vi "读取配置信息 (子VI).vi"(8 "error in (no error)":errorcluster caption="错误输入（无错误）") -> (0 "错误输出":errorcluster)   [LabVIEW 2022 SP3, in "流量计集成.lvlib"]
uses:
  <vilib>/Utility/config.llb/NI_LVConfig.lvlib
  <userlib>/_OpenG.lib/variantconfig/variantconfig.llb/openg_variant_configuration_file.lvlib
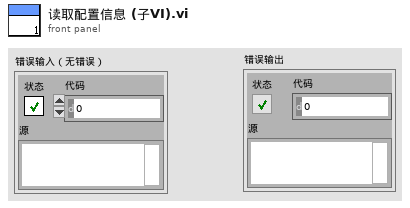
[diagram p1: front panel]
types:
  T1 = typedef "NI_LVConfig.lvlib/Config Data RefNum.ctl" = refnum<k1>
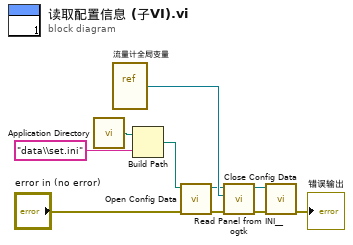
[diagram p0: block diagram]
diagram:
  n1 = call <vilib>:"Application Directory.vi"() -> ("Application Directory"=w4:path)
  n2 = vi-ref "流量计全局变量.vi"() -> (w9:refnum<vi>)
  n3 = Build Path(base path=w4, name or relative path="data\\set.ini" ("名称或相对路径")) -> (appended path=w3:path)
  n4 = call <vilib>:"Open Config Data.vi"("error in (no error)"="error in (no error)", "configuration file path"=w3) -> ("error out"=w6:errorcluster, "refnum"=w5:T1)  [unwired: 7 in, 1 out]
  n5 = call <userlib>:"Read Panel from INI__ogtk.vi"("error in (no error)"=w6, "VI ref"=w9, "refnum"=w5) -> ("error out"=w8:errorcluster, "refnum out"=w7:T1)  [unwired: 7 in]
  n6 = call <vilib>:"Close Config Data.vi"("error in (no error)"=w8, "refnum"=w7) -> ("error out"=→"错误输出":errorcluster)  [unwired: 8 in, 1 out]
